vi "EPTx Basic Example FPGA 1.0.vi"() -> ()   [LabVIEW 2020]
uses:
  <vilib>/Powertrain Controls/Device Drivers/Engine Position Tracking/EPTx/RevA/FPGA/Controls/EPTxTooth.ctl
  <vilib>/Powertrain Controls/Device Drivers/Engine Position Tracking/EPTx/RevA/FPGA/Controls/EPTxControl.ctl
  <vilib>/Powertrain Controls/Device Drivers/Engine Position Tracking/EPTx/RevA/FPGA/Controls/EPTxSignals.ctl
  <vilib>/Powertrain Controls/Device Drivers/Engine Position Tracking/EPTx/RevA/FPGA/Controls/EPTxSupervisor.ctl
  <vilib>/Powertrain Controls/Device Drivers/Engine Position Tracking/EPTx/RevA/FPGA/Controls/EPTxConfig.ctl
  <vilib>/Powertrain Controls/Device Drivers/Engine Position Tracking/EPTx/RevA/FPGA/Controls/EPTxPatternConfig.ctl
  <vilib>/Powertrain Controls/Device Drivers/Engine Position Tracking/EPTx/RevA/FPGA/Controls/Patterns.ctl
  <vilib>/Powertrain Controls/Device Drivers/Engine Position Tracking/EPTx/RevA/FPGA/Controls/EPTxDebug.ctl
  <vilib>/Powertrain Controls/Device Drivers/Engine Position Tracking/EPTx/RevA/FPGA/Controls/EPTxAAPControl.ctl
  <vilib>/Powertrain Controls/Device Drivers/Engine Position Tracking/EPTx/RevA/FPGA/Controls/EPTxSimulatorConfig.ctl
  <vilib>/Platform/TimedLoop/XDataNode/timing_clust.ctl
  <vilib>/Platform/TimedLoop/XDataNode/nitl_modes.ctl
  <vilib>/Platform/TimedLoop/XDataNode/wakeup.ctl
  <vilib>/rvi/Emulation/niFpgaSctlEmulationGetInTimedLoop.vi
  <vilib>/rvi/Emulation/niFpgaEmulationReportErrorSimple.vi
  <vilib>/rvi/Emulation/niFpgaGetClockAttributes.vi
  <vilib>/rvi/Emulation/niFpgaCriticalErrorInLSC.vi
  <vilib>/rvi/eio/common/nirviEmuTemplateMethod_errors.vi
  <vilib>/Platform/TimedLoop/XDataNode/XDataNode.xnode
  <vilib>/eio/EIONode/EIONode.xnode
  <vilib>/Platform/TimedLoop/XDataNode/XDNodeRunTimeDep.lvlib
  <vilib>/Powertrain Controls/Device Drivers/Engine Position Tracking/EPTx/RevA/FPGA/EPTx - RevA - FPGA.lvlib
panel:
  out "Cylinder_Number":u8
  in  "CylinderSig_6":T1 caption="簇" {"Cylinder6_H_F [CAD]" format="%.11g"; "Cylinder6_H_R [CAD]" format="%.11g"}
  in  "CylinderSig_5":T2 caption="簇" {"Cylinder5_H_F [CAD]" format="%.11g"; "Cylinder5_H_R [CAD]" format="%.11g"}
  in  "CylinderSig_4":T3 caption="簇" {"Cylinder4_H_F [CAD]" format="%.11g"; "Cylinder4_H_R [CAD]" format="%.11g"}
  in  "CylinderSig_3":T4 caption="簇" {"Cylinder3_H_F [CAD]" format="%.11g"; "Cylinder3_H_R [CAD]" format="%.11g"}
  in  "CylinderSig_2":T5 caption="簇" {"Cylinder2_H_F [CAD]" format="%.11g"; "Cylinder2_H_R [CAD]" format="%.11g"}
  in  "CylinderSig_1":T6 caption="簇" {"Cylinder1_H_F [CAD]" format="%.11g"; "Cylinder1_H_R [CAD]" format="%.11g"}
  in  "AAPControl_6str":T7
  in  "AAPControl_5str":T7
  in  "AAPControl_4str":T7
  in  "AAPControl_3str":T7
  in  "AAPControl_2str":T7
  in  "EPTxSimulatorConfig":T8
  in  "AAPControl_1str":T7
  out "EPTxDebug":T9
  in  "EPTxPatternConfig":T10 {"Pattern"."Aux_4" format="%#_16g"; "Pattern"."Aux_3" format="%#_16g"; "Pattern"."Aux_2" format="%#_16g"; "Pattern"."Aux_1" format="%#_16g"; "Pattern"."Primary" format="%#_16g"}
  out "Loop":u32
  in  "EPTxConfig":T12
  out "EPTxSupervisor":T13
  out "EPTxSignals":T14
  in  "EPTxControl":T15
  out "EPTxTooth":T16
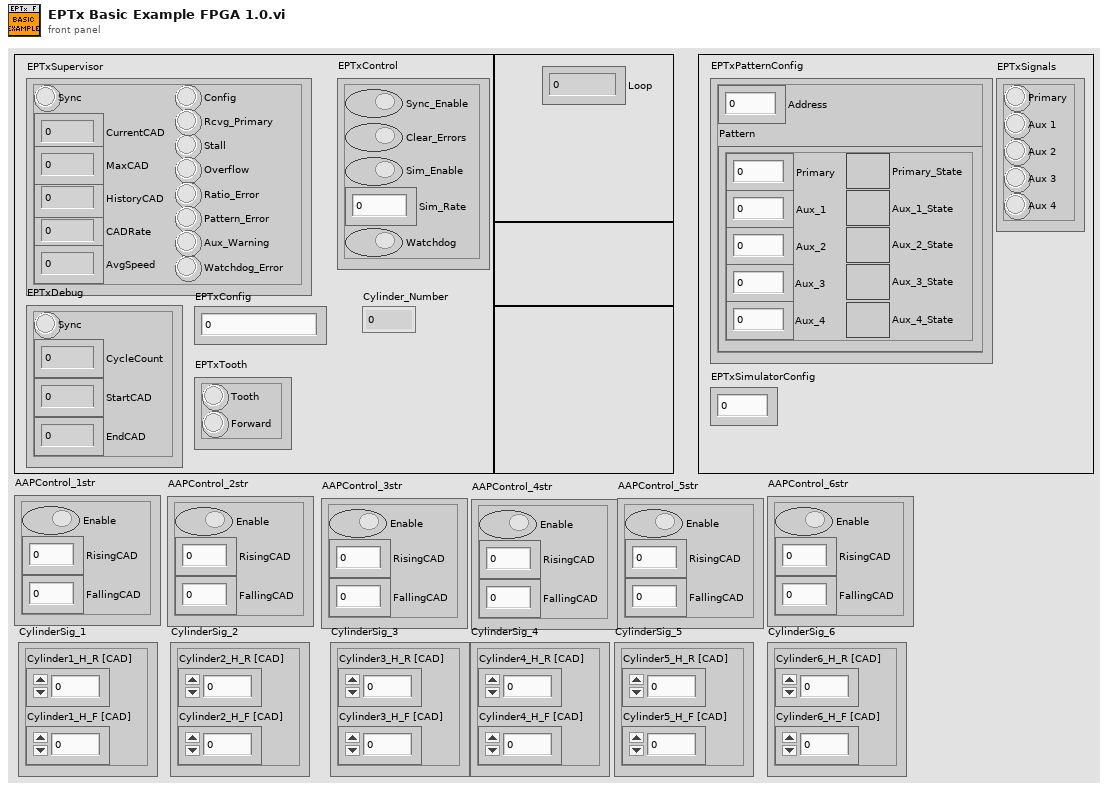
[diagram p1: front panel]
types:
  T1 = cluster{"Cylinder6_H_R [CAD]":fxp<+,18,11>, "Cylinder6_H_F [CAD]":fxp<+,18,11>}
  T2 = cluster{"Cylinder5_H_R [CAD]":fxp<+,18,11>, "Cylinder5_H_F [CAD]":fxp<+,18,11>}
  T3 = cluster{"Cylinder4_H_R [CAD]":fxp<+,18,11>, "Cylinder4_H_F [CAD]":fxp<+,18,11>}
  T4 = cluster{"Cylinder3_H_R [CAD]":fxp<+,18,11>, "Cylinder3_H_F [CAD]":fxp<+,18,11>}
  T5 = cluster{"Cylinder2_H_R [CAD]":fxp<+,18,11>, "Cylinder2_H_F [CAD]":fxp<+,18,11>}
  T6 = cluster{"Cylinder1_H_R [CAD]":fxp<+,18,11>, "Cylinder1_H_F [CAD]":fxp<+,18,11>}
  T7 = typedef "EPTx - RevA - FPGA.lvlib/EPTxAAPControl.ctl" = cluster{"Enable":bool, "RisingCAD":fxp<+,18,11>, "FallingCAD":fxp<+,18,11>}
  T8 = typedef "EPTx - RevA - FPGA.lvlib/EPTxSimulatorConfig.ctl" = u32
  T9 = typedef "EPTx - RevA - FPGA.lvlib/EPTxDebug.ctl" = cluster{"Sync":bool, "CycleCount":fxp<+,8,8>, "StartCAD":fxp<+,18,11>, "EndCAD":fxp<+,18,11>}
  T10 = typedef "EPTx - RevA - FPGA.lvlib/EPTxPatternConfig.ctl" = cluster{"Address":fxp<+,14,14>, "Pattern":T11}
  T11 = typedef "EPTx - RevA - FPGA.lvlib/Patterns.ctl" = cluster{"Primary":fxp<+,19,12>, "Primary_State":bool, "Aux_1":fxp<+,19,12>, "Aux_1_State":bool, "Aux_2":fxp<+,19,12>, "Aux_2_State":bool, "Aux_3":fxp<+,19,12>, "Aux_3_State":bool, "Aux_4":fxp<+,19,12>, "Aux_4_State":bool}
  T12 = typedef "EPTx - RevA - FPGA.lvlib/EPTxConfig.ctl" = u64
  T13 = typedef "EPTx - RevA - FPGA.lvlib/EPTxSupervisor.ctl" = cluster{"Sync":bool, "CurrentCAD":fxp<+,18,11>, "MaxCAD":fxp<+,11,11>, "HistoryCAD":fxp<+,11,11>, "CADRate":fxp<+,22,8>, "AvgSpeed":fxp<+,17,15>, "Config":bool, "Rcvg_Primary":bool, "Stall":bool, "Overflow":bool, "Ratio_Error":bool, "Pattern_Error":bool, "Aux_Warning":bool, "Watchdog_Error":bool}
  T14 = typedef "EPTx - RevA - FPGA.lvlib/EPTxSignals.ctl" = cluster{"Primary":bool, "Aux 1":bool, "Aux 2":bool, "Aux 3":bool, "Aux 4":bool}
  T15 = typedef "EPTx - RevA - FPGA.lvlib/EPTxControl.ctl" = cluster{"Sync_Enable":bool, "Clear_Errors":bool, "Sim_Enable":bool, "Sim_Rate":fxp<+,24,6>, "Watchdog":bool}
  T16 = typedef "EPTx - RevA - FPGA.lvlib/EPTxTooth.ctl" = cluster{"Tooth":bool, "Forward":bool}
  T17 = typedef "XDNodeRunTimeDep.lvlib/timing_clust.ctl" = cluster{"Expected End [f-1]":u64, "Actual End [f-1]":u64, "Finished Late? [f-1]":bool, "Expected End [i-1]":u64, "Actual End [i-1]":u64, "Finished Late? [i-1]":bool, "Expected Start [i]":u64, "Actual Start [i]":u64, "Expected Start [f]":u64, "Actual Start [f]":u64, "Source Name":string, "Structure Name":string, "Period":i64, "Deadline":i64, "Offset":i64, "Start":i64, "Priority":i32, "Timeout":i32, "Mode":T18, "Wakeup Reason":T19, "Error":errorcluster, "Source Type":string, "Secondary Source Type":string, "Global End Time":u64, "Global Start Time":u64, "Frame Duration":u64, "Iteration Duration":u64, "Assigned CPU":i32, "I/O Scan Engine Mode":u32}
  T18 = typedef "XDNodeRunTimeDep.lvlib/nitl_modes.ctl" = enum32{"No Change", "Process missed periods, maintain original phase", "Discard missed periods, maintain original phase", "Process missed periods, ignore original phase", "Discard missed periods, ignore original phase"}
  T19 = typedef "XDNodeRunTimeDep.lvlib/wakeup.ctl" = enum32{"Normal", "Aborted", "Asynchronous wakeup", "Timing source error", "Timed loop error", "Timeout"}
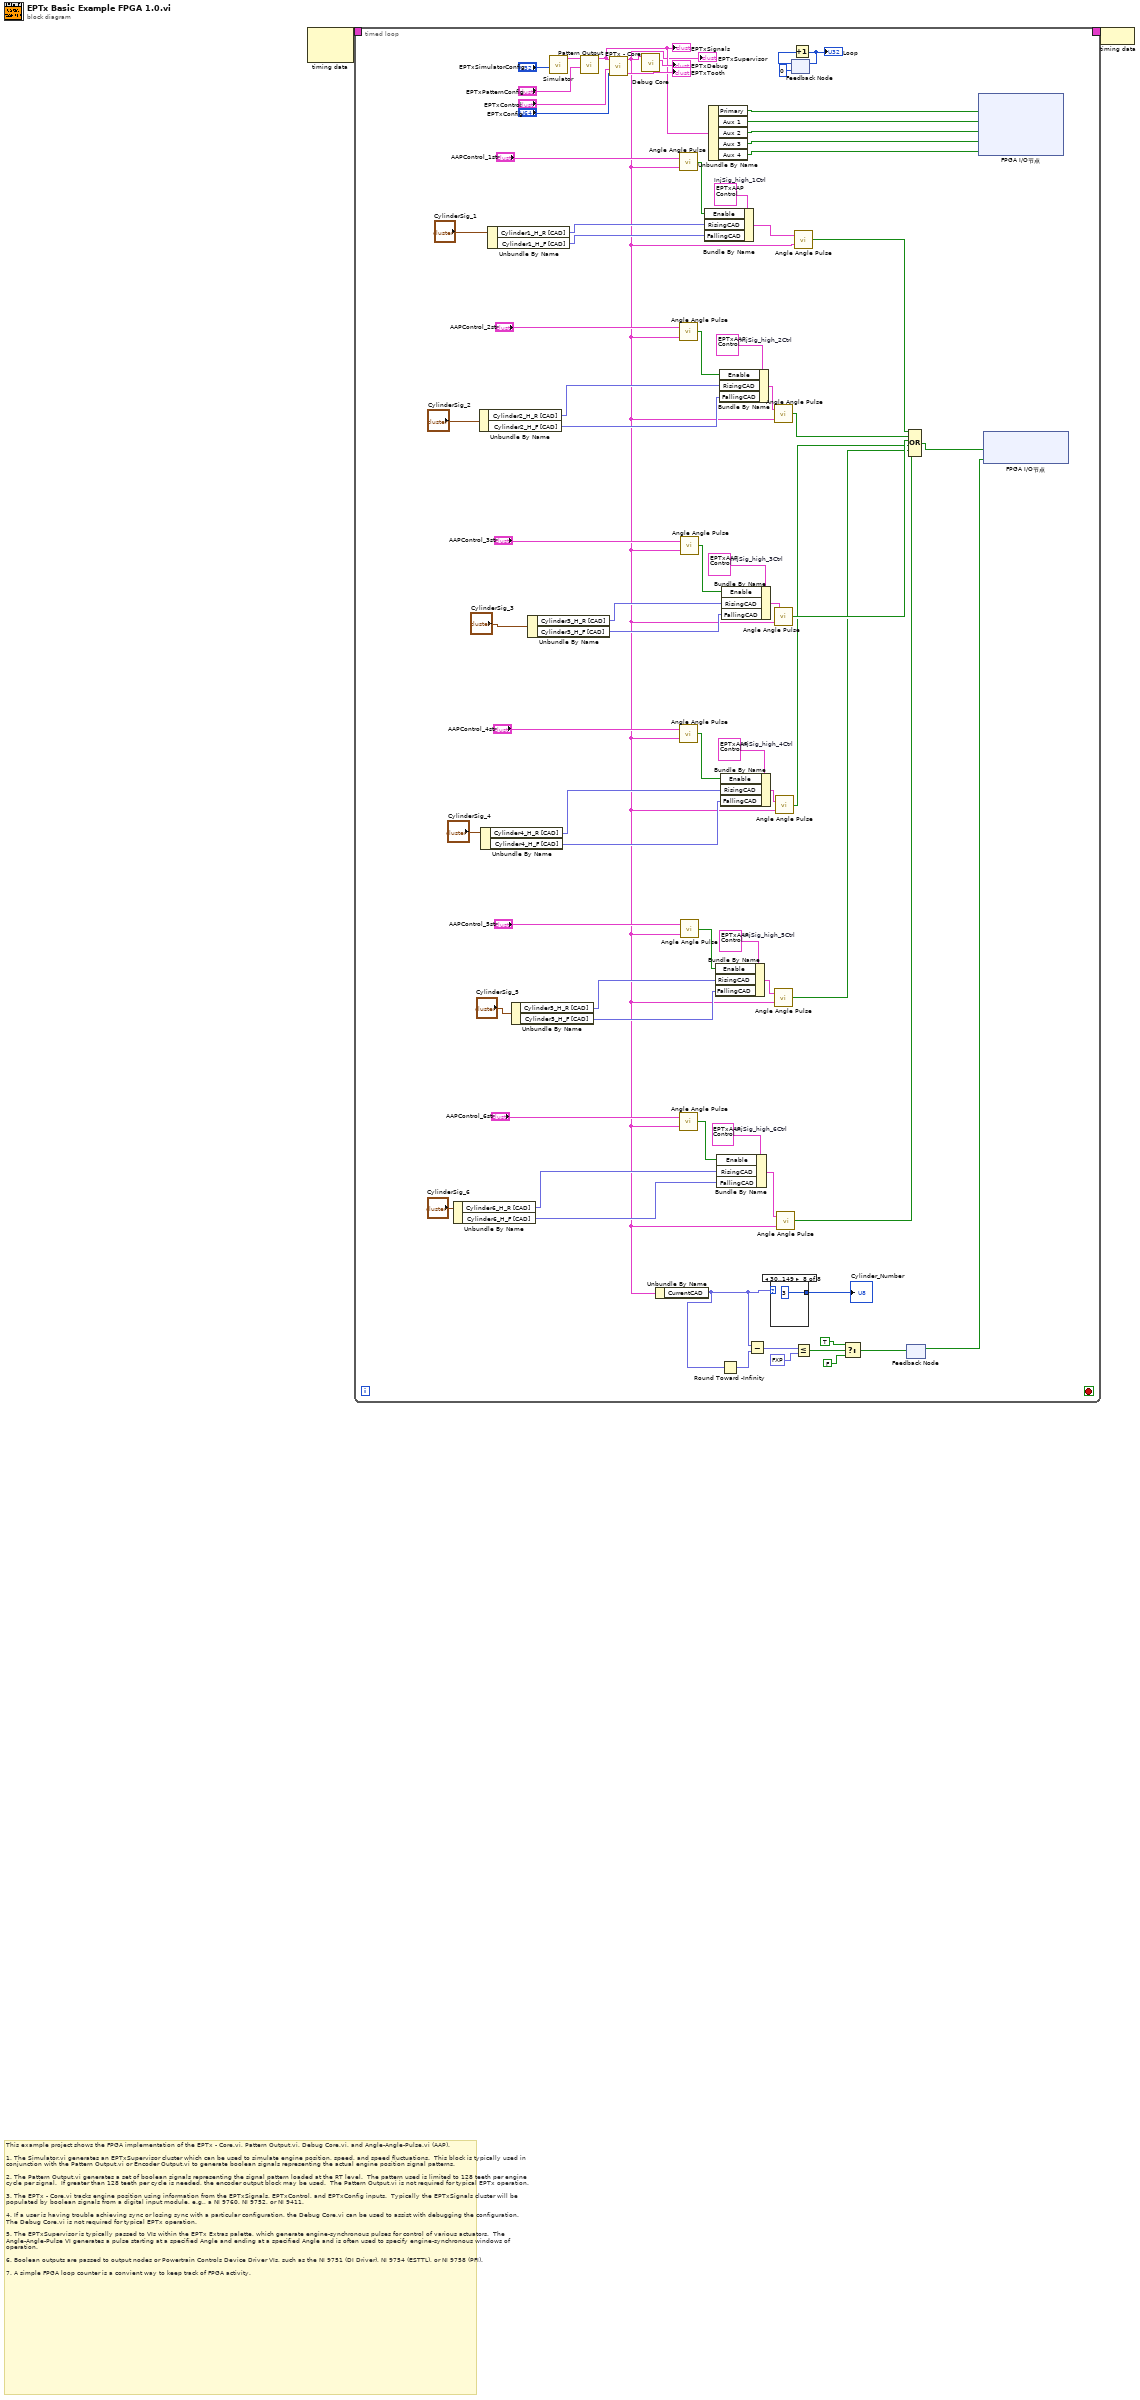
[diagram p0: block diagram]
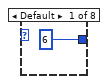
[diagram p2: hidden frame]
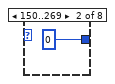
[diagram p3: hidden frame]
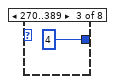
[diagram p4: hidden frame]
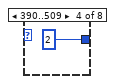
[diagram p5: hidden frame]
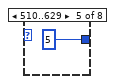
[diagram p6: hidden frame]
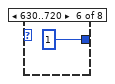
[diagram p7: hidden frame]
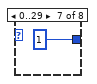
[diagram p8: hidden frame]
diagram:
  # "This example project shows the FPGA implementation of the EPTx - Core.vi, Pattern Output.vi, Debug Core.vi, and Angle-Angle-Pulse.vi (AAP).\n\n1. The Simulator.vi generates an EPTxSupervisor cluster which can be used to simulate engine position, speed, and speed fluctuations.  This block is typically used in conjunction with the Pattern Output.vi or Encoder Output.vi to generate boolean signals representing the actual engine position signal patterns.\n\n2. The Pattern Output.vi generates a set of boolean signals representing the signal pattern loaded at the RT level.  The pattern used is limited to 128 teeth per engine cycle per signal.  If greater than 128 teeth per cycle is needed, the encoder output block may be used.  The Pattern Output.vi is not required for typical EPTx operation.\n\n3. The EPTx - Core.vi tracks engine position using information from the EPTxSignals, EPTxControl, and EPTxConfig inputs.  Typically the EPTxSignals cluster will be populated by boolean signals from a digital input module, e.g., a NI 9760, NI 9752, or NI 9411.\n\n4. If a user is having trouble achieving sync or losing sync with a particular configuration, the Debug Core.vi can be used to assist with debugging the configuration.  The Debug Core.vi is not required for typical EPTx operation.\n\n5. The EPTxSupervisor is typically passed to VIs within the EPTx Extras palette, which generate engine-synchronous pulses for control of various actuators.  The Angle-Angle-Pulse VI generates a pulse starting at a specified Angle and ending at a specified Angle and is often used to specify engine-synchronous windows of operation.\n\n6. Boolean outputs are passed to output nodes or Powertrain Controls Device Driver VIs, such as the NI 9751 (DI Driver), NI 9754 (ESTTL), or NI 9758 (PFI).\n\n7. A simple FPGA loop counter is a convient way to keep track of FPGA activity."
  n1 = node-c288() -> (w2:T17)  [unwired: 2 in]
  n2 = timed-loop {
    timing: w2 -> [_]
    timing-out: [_] -> w1
    stop <- _ stop-if-true
    w47 = T7 {"Enable"=FALSE, "RisingCAD"=0.0, "FallingCAD"=0.0}  # InjSig_high_6Ctrl
    w49 = T7 {"Enable"=FALSE, "RisingCAD"=0.0, "FallingCAD"=0.0}  # InjSig_high_5Ctrl
    w51 = T7 {"Enable"=FALSE, "RisingCAD"=0.0, "FallingCAD"=0.0}  # InjSig_high_4Ctrl
    w52 = T7 {"Enable"=FALSE, "RisingCAD"=0.0, "FallingCAD"=0.0}  # InjSig_high_3Ctrl
    w54 = T7 {"Enable"=FALSE, "RisingCAD"=0.0, "FallingCAD"=0.0}  # InjSig_high_2Ctrl
    w55 = T7 {"Enable"=FALSE, "RisingCAD"=0.0, "FallingCAD"=0.0}  # InjSig_high_1Ctrl
    n3 = Unbundle By Name("CylinderSig_6") -> ("Cylinder6_H_R [CAD]"=w22:fxp<+,18,11>, "Cylinder6_H_F [CAD]"=w21:fxp<+,18,11>)
    n4 = Unbundle By Name("CylinderSig_2") -> ("Cylinder2_H_R [CAD]"=w25:fxp<+,18,11>, "Cylinder2_H_F [CAD]"=w24:fxp<+,18,11>)
    n5 = Unbundle By Name("CylinderSig_4") -> ("Cylinder4_H_R [CAD]"=w28:fxp<+,18,11>, "Cylinder4_H_F [CAD]"=w27:fxp<+,18,11>)
    n6 = Unbundle By Name("CylinderSig_1") -> ("Cylinder1_H_R [CAD]"=w38:fxp<+,18,11>, "Cylinder1_H_F [CAD]"=w37:fxp<+,18,11>)
    n7 = Unbundle By Name("CylinderSig_5") -> ("Cylinder5_H_R [CAD]"=w32:fxp<+,18,11>, "Cylinder5_H_F [CAD]"=w31:fxp<+,18,11>)
    n8 = Unbundle By Name("CylinderSig_3") -> ("Cylinder3_H_R [CAD]"=w35:fxp<+,18,11>, "Cylinder3_H_F [CAD]"=w34:fxp<+,18,11>)
    n9 = call <vilib>:"Simulator.vi"("EPTxSimulatorConfig"="EPTxSimulatorConfig") -> ("EPTxSupervisor"=w70:T13)  [unwired: 10 in]
    n10 = call <vilib>:"Pattern Output.vi"("EPTxPatternConfig"="EPTxPatternConfig", "EPTxSupervisor"=w70) -> ("PatternOutput"=w67:T14)  [unwired: 9 in]
    "EPTxSignals" <- w67
    n11 = call <vilib>:"EPTx - Core.vi"("EPTxConfig"="EPTxConfig", "EPTxControl"="EPTxControl", "EPTxSignals"=w67) -> ("EPTxTooth"=→"EPTxTooth":T16, "EPTxSupervisor"=w12:T13)  [unwired: 7 in]
    "EPTxSupervisor" <- w12
    n12 = call <vilib>:"Debug Core.vi"("EPTxSupervisor"=w12) -> ("EPTxDebug"=→"EPTxDebug":T9)  [unwired: 10 in]
    n13 = Unbundle By Name(w12) -> ("CurrentCAD"=w11:fxp<+,18,11>)
    n14 = call <vilib>:"Angle Angle Pulse.vi"("EPTxSupervisor"=w12, "AAPControl"="AAPControl_1str") -> ("AAP"=w45:bool)
    n15 = call <vilib>:"Angle Angle Pulse.vi"("EPTxSupervisor"=w12, "AAPControl"="AAPControl_2str") -> ("AAP"=w44:bool)
    n16 = call <vilib>:"Angle Angle Pulse.vi"("EPTxSupervisor"=w12, "AAPControl"="AAPControl_4str") -> ("AAP"=w42:bool)
    n17 = call <vilib>:"Angle Angle Pulse.vi"("EPTxSupervisor"=w12, "AAPControl"="AAPControl_6str") -> ("AAP"=w40:bool)
    n18 = call <vilib>:"Angle Angle Pulse.vi"("EPTxSupervisor"=w12, "AAPControl"="AAPControl_3str") -> ("AAP"=w43:bool)
    n19 = call <vilib>:"Angle Angle Pulse.vi"("EPTxSupervisor"=w12, "AAPControl"="AAPControl_5str") -> ("AAP"=w41:bool)
    n20 = Bundle By Name(cluster=w55, "Enable"=w45, "RisingCAD"=w38, "FallingCAD"=w37) -> (w56:T7)
    n21 = Unbundle By Name(w67) -> ("Primary"=w66:bool, "Aux 1"=w65:bool, "Aux 2"=w64:bool, "Aux 3"=w63:bool, "Aux 4"=w62:bool)
    n22 = Bundle By Name(cluster=w49, "Enable"=w41, "RisingCAD"=w32, "FallingCAD"=w31) -> (w48:T7)
    n23 = Bundle By Name(cluster=w47, "Enable"=w40, "RisingCAD"=w22, "FallingCAD"=w21) -> (w46:T7)
    n24 = Bundle By Name(cluster=w54, "Enable"=w44, "RisingCAD"=w25, "FallingCAD"=w24) -> (w53:T7)
    n25 = Bundle By Name(cluster=w51, "Enable"=w42, "RisingCAD"=w28, "FallingCAD"=w27) -> (w50:T7)
    n26 = Round Toward -Infinity(1:w11) -> (0:w10:fxp<+,11,11>)
    n27 = Bundle By Name(cluster=w52, "Enable"=w43, "RisingCAD"=w35, "FallingCAD"=w34) -> (w30:T7)
    n28 = Subtract(x=w11, y=w10) -> (x-y=w9:fxp<+/-,19,12>)
    n29 = case shown="30..149" w11 {
      tunnel: [u8 6 u8 0 u8 4 u8 2 u8 5 u8 1 u8 1 u8 3] -> w13
      frame Default {
      }
      frame 150..269 {
      }
      frame 270..389 {
      }
      frame 390..509 {
      }
      frame 510..629 {
      }
      frame 630..720 {
      }
      frame 0..29 {
      }
      frame 30..149 {
      }
    }
    "Cylinder_Number" <- w13
    n30 = call <vilib>:"Angle Angle Pulse.vi"("EPTxSupervisor"=w12, "AAPControl"=w53) -> ("AAP"=w19:bool)
    n31 = call <vilib>:"Angle Angle Pulse.vi"("EPTxSupervisor"=w12, "AAPControl"=w30) -> ("AAP"=w18:bool)
    n32 = call <vilib>:"Angle Angle Pulse.vi"("EPTxSupervisor"=w12, "AAPControl"=w48) -> ("AAP"=w16:bool)
    n33 = call <vilib>:"Angle Angle Pulse.vi"("EPTxSupervisor"=w12, "AAPControl"=w50) -> ("AAP"=w17:bool)
    n34 = call <vilib>:"Angle Angle Pulse.vi"("EPTxSupervisor"=w12, "AAPControl"=w46) -> ("AAP"=w15:bool)
    n35 = feedback #1(u32 0) -> (w75:u32)
    n36 = Increment(x=w75) -> (x+1=w76:u32)
    "Loop" <- w76
    n37 = feedback-in #1(w76) -> ()
    n38 = call <vilib>:"Angle Angle Pulse.vi"("EPTxSupervisor"=w12, "AAPControl"=w56) -> ("AAP"=w20:bool)
    n39 = Less Or Equal?(x=w9, y=fxp<+/-,19,12> 0.5) -> (x <= y?=w7:bool)
    n40 = Select(t=TRUE, s=w7, f=FALSE) -> (s? t:f=w4:bool)
    n41 = feedback-in #2(w4) -> ()
    n42 = feedback #2() -> (w3:bool)  [unwired: 1 in]
    n43 = Compound Arithmetic op=OR ("复合运算")(w20, w19, w18, w17, w16, w15) -> (w14:bool)
    n44 = xnode "FPGA I/O节点"("Connector0/DIO4"=w66, "Connector0/DIO5"=w65, "Connector0/DIO6"=w64, "Connector0/DIO7"=w63, "Connector0/DIO8"=w62) -> ()  [unwired: 5 in, 5 out]
    n45 = xnode "FPGA I/O节点"("Connector1/DIO0"=w14, "Connector1/DIO1"=w3) -> ()  [unwired: 2 in, 2 out]
  }
  n46 = node-c288(w1) -> ()
